vi "Get ID.vi"(8 "error in (no error)":errorcluster, 11 "Connection in":refnum<class "Connection.lvclass">) -> (0 "error out":errorcluster, 2 "ID":i32, 3 "Connection out":refnum<class "Connection.lvclass">)   [LabVIEW 2020, in "Parallel Block.lvlib" / "Connection.lvclass"]
uses:
  Connection.lvclass
  Connection.lvclass/Connection.ctl
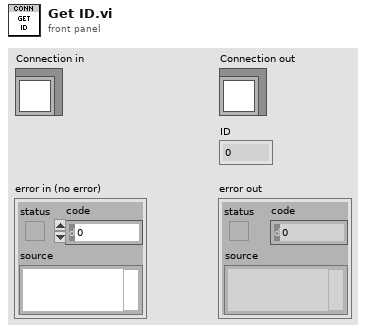
[diagram p1: front panel]
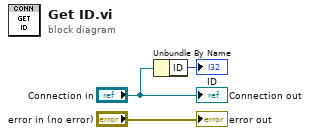
[diagram p0: block diagram]
diagram:
  n1 = Unbundle By Name("Connection in") -> ("ID"=→"ID":i32)
  "error out" <- "error in (no error)"
  "Connection out" <- "Connection in"
